vi "LEDs.vi"() -> ()   [LabVIEW 2014]
uses:
  Utility/Labview GEA2 Toolkit v2.1/type defs/Data In.ctl
  Utility/Labview GEA2 Toolkit v2.1/library/GEA2_Toolkit.lvlib
panel:
  out "Message":string
  out "Channel_Cycle_Unmapped":bool
  out "Channel_Off":bool
  out "Z310 - E-Wash":bool
  out "Z309 - Auto Soak":bool
  out "Z308 - Fabric Soft":bool
  out "Z307 - Extra Rinse":bool
  out "Z306 - Delay Wash":bool
  out "Z305 - My Cycles":bool
  out "Z304 - Tomato":bool
  out "Z303 - Oily":bool
  out "Z302 - Grease":bool
  out "Z301 - Dirt":bool
  out "Unused3":bool
  out "Unused2":bool
  out "Unused1":bool
  out "Unused0":bool
  out "Z159 - Rinse":bool
  out "Z158 - Spin":bool
  out "Z157 - Done":bool
  out "Z151 - Wash":bool
  out "Z150 - Soak":bool
  out "Z149 - Delay":bool
  out "Z148":bool
  out "Z146":bool
  out "Z147- Controls":bool
  out "Z145 - Lid Lock":bool
  out "Z144 - Good":bool
  out "Z143":bool
  out "Z142":bool
  out "Z141 - Better":bool
  out "Z140":bool
  out "Z139":bool
  out "Z138":bool
  out "Z137":bool
  out "Z136":bool
  out "Z135":bool
  out "Z134":bool
  out "Z133":bool
  out "Z132":bool
  out "Z131":bool
  out "Z130 - Pause":bool
  out "Z129":bool
  out "Z128":bool
  out "Z127":bool
  out "Z164 - No Spin":bool
  out "Z163 - Low":bool
  out "Z162 - Medium":bool
  out "Z161 - High":bool
  out "Z160 - Extra High":bool
  out "Z156 - Extra Light":bool
  out "Z155 - Light":bool
  out "Z154 - Normal":bool
  out "Z153 - Heavy":bool
  out "Z152 - Extra Heavy":bool
  out "Z126":bool
  out "Z125":bool
  out "Z124":bool
  out "Z123":bool
  out "Z122 - Tap Cold":bool
  out "Z121 - Cold":bool
  out "Z120 - Cool":bool
  out "Z119 - Colors":bool
  out "Z118 - Warm":bool
  out "Z117 - Hot":bool
  out "Z115":bool
  out "Z102":bool
  out "Z103":bool
  out "Z104":bool
  out "Z105":bool
  out "Z106":bool
  out "Z107":bool
  out "Z108":bool
  out "Z109":bool
  out "Z110":bool
  out "Z111":bool
  out "Z112":bool
  out "Z113":bool
  out "Z114":bool
  out "Z116":bool
  out "Z101":bool
  # "0"
  # "Knob"
  # "Not Used"
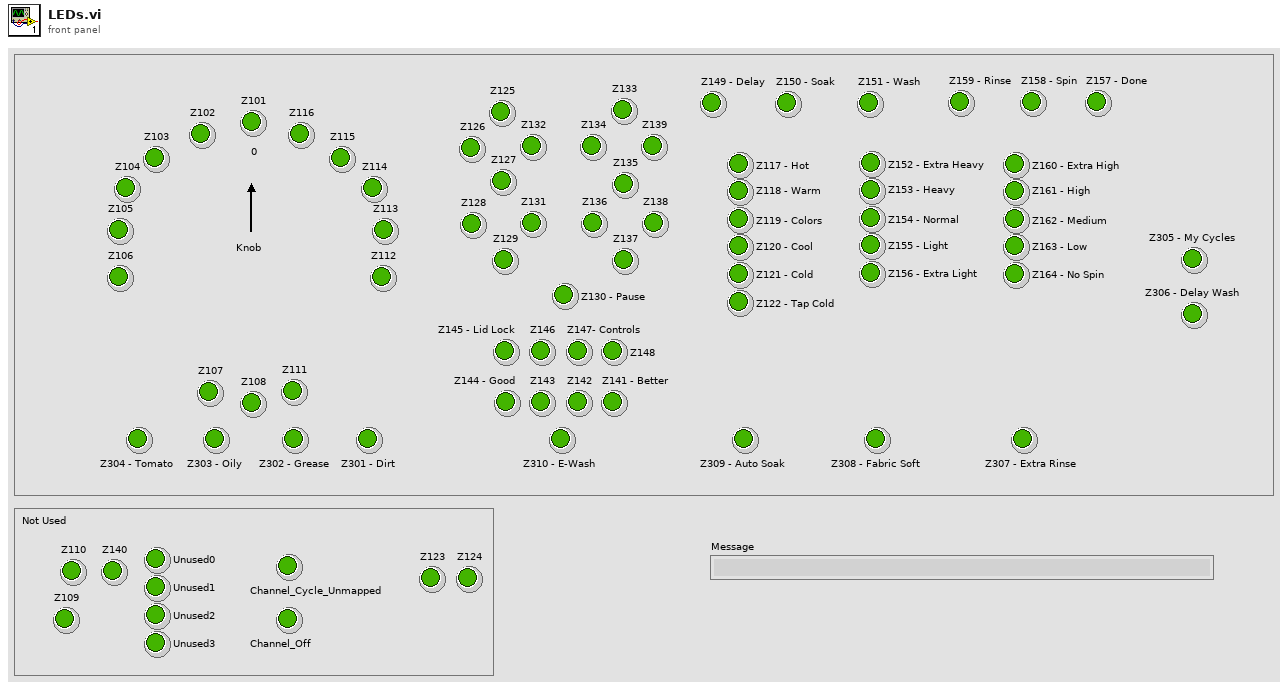
[diagram p1: front panel]
types:
  T1 = typedef "GEA2_Toolkit.lvlib/Data In.ctl" = cluster{"Source":u8, "Destination":u8, "Command":u8, "Message":string}
  T2 = typedef "GEA2_Toolkit.lvlib/Data Out.ctl" = cluster{"Source":u8, "Destination":u8, "Command":u8, "Length":u8, "CRC":u16, "Message":string}
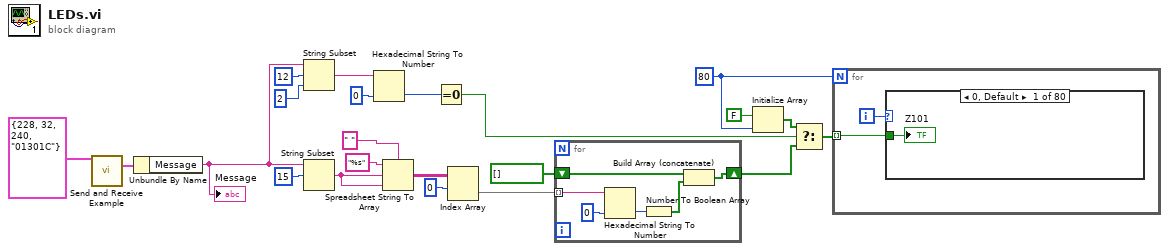
[diagram p0: block diagram]
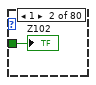
[diagram p2: hidden frame]
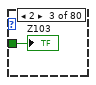
[diagram p3: hidden frame]
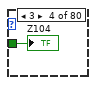
[diagram p4: hidden frame]
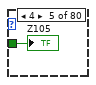
[diagram p5: hidden frame]
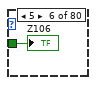
[diagram p6: hidden frame]
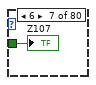
[diagram p7: hidden frame]
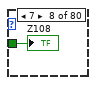
[diagram p8: hidden frame]
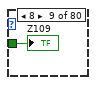
[diagram p9: hidden frame]
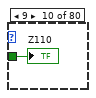
[diagram p10: hidden frame]
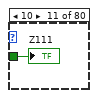
[diagram p11: hidden frame]
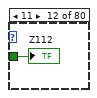
[diagram p12: hidden frame]
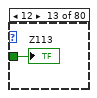
[diagram p13: hidden frame]
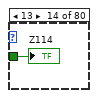
[diagram p14: hidden frame]
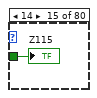
[diagram p15: hidden frame]
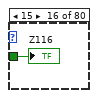
[diagram p16: hidden frame]
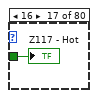
[diagram p17: hidden frame]
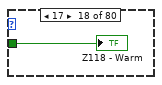
[diagram p18: hidden frame]
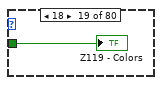
[diagram p19: hidden frame]
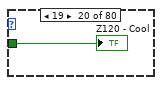
[diagram p20: hidden frame]
diagram:
  w3 = 80
  n1 = call "Send and Receive Example.vi"("Input Data"=T1 {"Source"=228, "Destination"=32, "Command"=240, "Message"="01301C"}) -> ("Coverted Data Out"=w21:T2)  [unwired: 12 in, 2 out]
  n2 = Unbundle By Name(w21) -> ("Message"=w11:string)
  "Message" <- w11
  n3 = String Subset(string=w11, offset (0)=12, length (rest)=2 ("length (rest)")) -> (substring=w10:string)
  n4 = String Subset(string=w11, offset (0)=15) -> (substring=w14:string)  [unwired: 1 in]
  n5 = Hexadecimal String To Number(string=w10, default (0uL)=u32 0 ("default (0 U32)")) -> (number=w8:u32)  [unwired: 1 in, 1 out]
  n6 = Spreadsheet String To Array(delimiter (Tab)=" ", format string="%s", spreadsheet string=w14, array type (2D Dbl)=w14) -> (array=w18:string[][])
  n7 = Equal To 0?(x=w8) -> (x = 0?=w7:bool)
  n8 = Index Array(array=w18, index (row)=0) -> (element=w15:string[])  [unwired: 1 in]
  n9 = for {
    tunnel: w15 -> [w28] mode=indexing
    shift-right: [w24] -> w5
    shift-left: bool[] [] -> [w26]
    n10 = Hexadecimal String To Number(string=w28, default (0uL)=u8 0) -> (number=w27:u8)  [unwired: 1 in, 1 out]
    n11 = Number To Boolean Array(number=w27) -> (Boolean array=w25:bool[])
    n12 = Build Array (concatenate)(w26, w25) -> (w24:bool[])
  }
  n13 = Initialize Array(FALSE, w3) -> (w2:bool[])
  n14 = Select(t=w2, s=w7, f=w5) -> (s? t:f=w6:bool[])
  n15 = for {
    N: w3 -> [_]
    tunnel: w6 -> [w29] mode=indexing
    i -> [w30]
    n16 = case shown="0, Default" w30 {
      tunnel: w29 -> [w31 w32 w33 w34 w35 w36 w37 w38 w39 w40 w41 w42 w43 w44 w45 w46 w47 w48 w49 w50 w51 w52 w53 w54 w55 w56 w57 w58 w59 w60 w61 w62 w63 w64 w65 w66 w67 w68 w69 w70 w71 w72 w73 w74 w75 w76 w77 w78 w79 w80 w81 w82 w83 w84 w85 w86 w87 w88 w89 w90 w91 w92 w93 w94 w95 w96 w97 w98 w99 w100 w101 w102 w103 w104 w105 w106 w107 w108 w109 w110]
      frame 0, Default {
        "Z101" <- w31
      }
      frame 1 {
        "Z102" <- w32
      }
      frame 2 {
        "Z103" <- w33
      }
      frame 3 {
        "Z104" <- w34
      }
      frame 4 {
        "Z105" <- w35
      }
      frame 5 {
        "Z106" <- w36
      }
      frame 6 {
        "Z107" <- w37
      }
      frame 7 {
        "Z108" <- w38
      }
      frame 8 {
        "Z109" <- w39
      }
      frame 9 {
        "Z110" <- w40
      }
      frame 10 {
        "Z111" <- w41
      }
      frame 11 {
        "Z112" <- w42
      }
      frame 12 {
        "Z113" <- w43
      }
      frame 13 {
        "Z114" <- w44
      }
      frame 14 {
        "Z115" <- w45
      }
      frame 15 {
        "Z116" <- w46
      }
      frame 16 {
        "Z117 - Hot" <- w47
      }
      frame 17 {
        "Z118 - Warm" <- w48
      }
      frame 18 {
        "Z119 - Colors" <- w49
      }
      frame 19 {
        "Z120 - Cool" <- w50
      }
      frame 20 {
        "Z121 - Cold" <- w51
      }
      frame 21 {
        "Z122 - Tap Cold" <- w52
      }
      frame 22 {
        "Z123" <- w53
      }
      frame 23 {
        "Z124" <- w54
      }
      frame 24 {
        "Z125" <- w55
      }
      frame 25 {
        "Z126" <- w56
      }
      frame 26 {
        "Z127" <- w57
      }
      frame 27 {
        "Z128" <- w58
      }
      frame 28 {
        "Z129" <- w59
      }
      frame 29 {
        "Z130 - Pause" <- w60
      }
      frame 30 {
        "Z131" <- w61
      }
      frame 31 {
        "Z132" <- w62
      }
      frame 32 {
        "Z133" <- w63
      }
      frame 33 {
        "Z134" <- w64
      }
      frame 34 {
        "Z135" <- w65
      }
      frame 35 {
        "Z136" <- w66
      }
      frame 36 {
        "Z137" <- w67
      }
      frame 37 {
        "Z138" <- w68
      }
      frame 38 {
        "Z139" <- w69
      }
      frame 39 {
        "Z140" <- w70
      }
      frame 40 {
        "Z141 - Better" <- w71
      }
      frame 41 {
        "Z142" <- w72
      }
      frame 42 {
        "Z143" <- w73
      }
      frame 43 {
        "Z144 - Good" <- w74
      }
      frame 44 {
        "Z145 - Lid Lock" <- w75
      }
      frame 45 {
        "Z146" <- w76
      }
      frame 46 {
        "Z147- Controls" <- w77
      }
      frame 47 {
        "Z148" <- w78
      }
      frame 48 {
        "Z149 - Delay" <- w79
      }
      frame 49 {
        "Z150 - Soak" <- w80
      }
      frame 50 {
        "Z151 - Wash" <- w81
      }
      frame 51 {
        "Z152 - Extra Heavy" <- w82
      }
      frame 52 {
        "Z153 - Heavy" <- w83
      }
      frame 53 {
        "Z154 - Normal" <- w84
      }
      frame 54 {
        "Z155 - Light" <- w85
      }
      frame 55 {
        "Z156 - Extra Light" <- w86
      }
      frame 56 {
        "Z157 - Done" <- w87
      }
      frame 57 {
        "Z158 - Spin" <- w88
      }
      frame 58 {
        "Z159 - Rinse" <- w89
      }
      frame 59 {
        "Z160 - Extra High" <- w90
      }
      frame 60 {
        "Z161 - High" <- w91
      }
      frame 61 {
        "Z162 - Medium" <- w92
      }
      frame 62 {
        "Z163 - Low" <- w93
      }
      frame 63 {
        "Z164 - No Spin" <- w94
      }
      frame 64 {
        "Unused0" <- w95
      }
      frame 65 {
        "Unused1" <- w96
      }
      frame 66 {
        "Unused2" <- w97
      }
      frame 67 {
        "Unused3" <- w98
      }
      frame 68 {
        "Z301 - Dirt" <- w99
      }
      frame 69 {
        "Z302 - Grease" <- w100
      }
      frame 70 {
        "Z303 - Oily" <- w101
      }
      frame 71 {
        "Z304 - Tomato" <- w102
      }
      frame 72 {
        "Z305 - My Cycles" <- w103
      }
      frame 73 {
        "Z306 - Delay Wash" <- w104
      }
      frame 74 {
        "Z307 - Extra Rinse" <- w105
      }
      frame 75 {
        "Z308 - Fabric Soft" <- w106
      }
      frame 76 {
        "Z309 - Auto Soak" <- w107
      }
      frame 77 {
        "Z310 - E-Wash" <- w108
      }
      frame 78 {
        "Channel_Off" <- w109
      }
      frame 79 {
        "Channel_Cycle_Unmapped" <- w110
      }
    }
  }
